vi "Toggle Test.vi"() -> ()   [LabVIEW 2011]
panel:
  out "Boolean 4":bool
  in  "Boolean 3":bool
  out "Boolean 2":bool
  in  "Boolean":bool
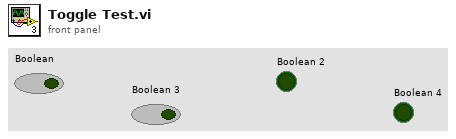
[diagram p1: front panel]
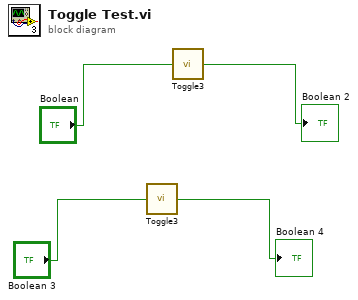
[diagram p0: block diagram]
diagram:
  n1 = call "Toggle3.vi"("In"="Boolean 3") -> ("Out"=→"Boolean 4":bool)
  n2 = call "Toggle3.vi"("In"="Boolean") -> ("Out"=→"Boolean 2":bool)
